vi "LabVIEW back up 05 10.vi"() -> ()   [LabVIEW 2015]
uses:
  <vilib>/DAQmx/read.llb/DAQmx Read (Analog 1D DBL NChan 1Samp).vi
  <vilib>/DAQmx/create/channels.llb/DAQmx Create Channel (AI-Voltage-Basic).vi
  <vilib>/DAQmx/miscellaneous.llb/DAQmx Fill In Error Info.vi
  Program Files/neMESYS_SDK/neMESYS LabVIEW Kit/neMESYS LabVIEW Integration Kit.lvlib
  Conor/Temp CN7500/Omega CN7500/Omega CN7500.lvlib
panel:
  in  "Empty Syringe Shut Down":bool
  out "Safety Shut Down Temp (oC)":dbl
  out "Safety Shut Down Pressure (barg)":dbl
  out "Text Read From Clipboard 5":string
  out "Read error out 5":errorcluster
  out "Write Set Point Status 2":string
  out "Error Out 5":i32
  out "Write error out 5":errorcluster
  out "Temperature":dynamicdata(graph)
  in  "Set Point (oC)":dbl
  out "Actual Temp (oC)":dbl
  out "Temp Set Point (oC)":dbl
  in  "Temperature Set Point":bool
  in  "Change New Set Points":bool
  in  "Read Set Points":bool
  in  "Test Gas Communication":bool
  out "Text Read From Clipboard":string
  out "Read error out":errorcluster
  out "Test Status":string
  out "Error Out":i32
  out "Write error out":errorcluster
  out "Text Read From Clipboard 4":string
  out "Read error out 4":errorcluster
  out "Write Set Point Status":string
  out "Error Out 4":i32
  out "Write error out 4":errorcluster
  in  "Set Point 1 (NmL/min)":dbl
  in  "Set Point 2 (NmL/min)":dbl
  in  "Set Point 3 (NmL/min)":dbl
  out "Flow Span of All Controlers (NmL/min)":dbl
  in  "Set Point 4 (NmL/min)":dbl
  out "Set Point Function":string
  out "Text Read From Clipboard 3":string
  out "Read error out 3":errorcluster
  out "Read Set Point Status":string
  out "Error Out 3":i32
  out "Write error out 3":errorcluster
  out "Text Read From Clipboard 2":string
  out "Read error out 2":errorcluster
  out "Read Flow Status":string
  out "Gas Flow 1 NmL/min":dbl
  out "Gas Flow 2 NmL/min":dbl
  out "Gas Flow 3 NmL/min":dbl
  out "Gas Flow 4 NmL/min":dbl
  out "Gas Flow rate":dynamicdata(graph)
  out "First waste string":string
  out "Rest of string 1":string
  out "First Number":string
  out "Rest of string 2":string
  out "Second Number 2":string
  out "Rest of string 3":string
  out "Third Number 3":string
  out "Rest of string 4":string
  out "Fourth Number 3":string
  out "Rest of string 5":string
  out "Error Out 2":i32
  out "Write error out 2":errorcluster
  in  "Refill 4":bool
  in  "Refill 3":bool
  in  "Refill 2":bool
  in  "Refill 1":bool
  in  "Empty 4":bool
  in  "Empty 3":bool
  in  "Empty 2":bool
  in  "Empty 1":bool
  in  "Calibrate 4":bool
  in  "Calibrate 3":bool
  in  "Calibrate 2":bool
  in  "Calibrate 1":bool
  in  "Stop Dose 4":bool
  in  "Stop Dose 3":bool
  in  "Stop Dose 2":bool
  in  "Stop Dose 1":bool
  in  "Set Level":bool
  in  "Dose Volume":bool
  in  "Generate Flow":bool
  in  "Dose Volume 4":dbl
  in  "Dose Volume 3":dbl
  in  "Dose Volume 2":dbl
  in  "Dose Volume 1":dbl
  in  "Set Level 4":dbl
  in  "Set Level 3":dbl
  in  "Set Level 2":dbl
  in  "Set Level 1":dbl
  in  "Set Flowrate 4":dbl
  in  "Set Flowrate 3":dbl
  in  "Set Flowrate 2":dbl
  in  "Set Flowrate 1":dbl
  out "Syringe Level 4":dbl
  out "Syringe Level 3":dbl
  out "Syringe Level 2":dbl
  out "Syringe Level 1":dbl
  out "Actual Flowrate 4":dbl
  out "Actual Flowrate 3":dbl
  out "Actual Flowrate 2":dbl
  out "Actual Flowrate 1":dbl
  out "Volume unit 1":string
  out "Level Max 1":dbl
  out "Flow unit 1":string
  out "Flow Max 1":dbl
  out "Number of Dosing Units":dbl
  out "Pressure 4 (barg)":dbl
  out "Pressure 3 (barg)":dbl
  out "Pressure 2 (barg)":dbl
  out "Pressure 1 (barg)":dbl
  out "Pressure 4 (PSIG)":dbl
  out "Pressure 3 (PSIG)":dbl
  out "Pressure 2 (PSIG)":dbl
  out "Pressure 1 (PSIG)":dbl
  out "Slope 4":dbl
  out "Slope 3":dbl
  out "Slope 2":dbl
  out "Intercept 4":dbl
  out "Intercept  3":dbl
  out "Intercept 2":dbl
  out "Intercept 1":dbl
  out "Slope 1":dbl
  out "Calibration File: 2":path
  in  "Clear":bool
  out "Calculated Pressure":dbl[][](graph)
  in  "stop":bool
  # "Volume and Flow units are fixed in this VI \nand we assume all syringes are identical\nBut making them a selection is easy if needed"
  # "Nemesys Pumps"
  # "Pressure Sensors"
  # "Sensor Calibration (y=psi, x=Volts) \nCalibration File is Pcal"
  # "Brooks software must be running for this to work!!!"
  # "Gas MFC"
  # "Temperature Controller"
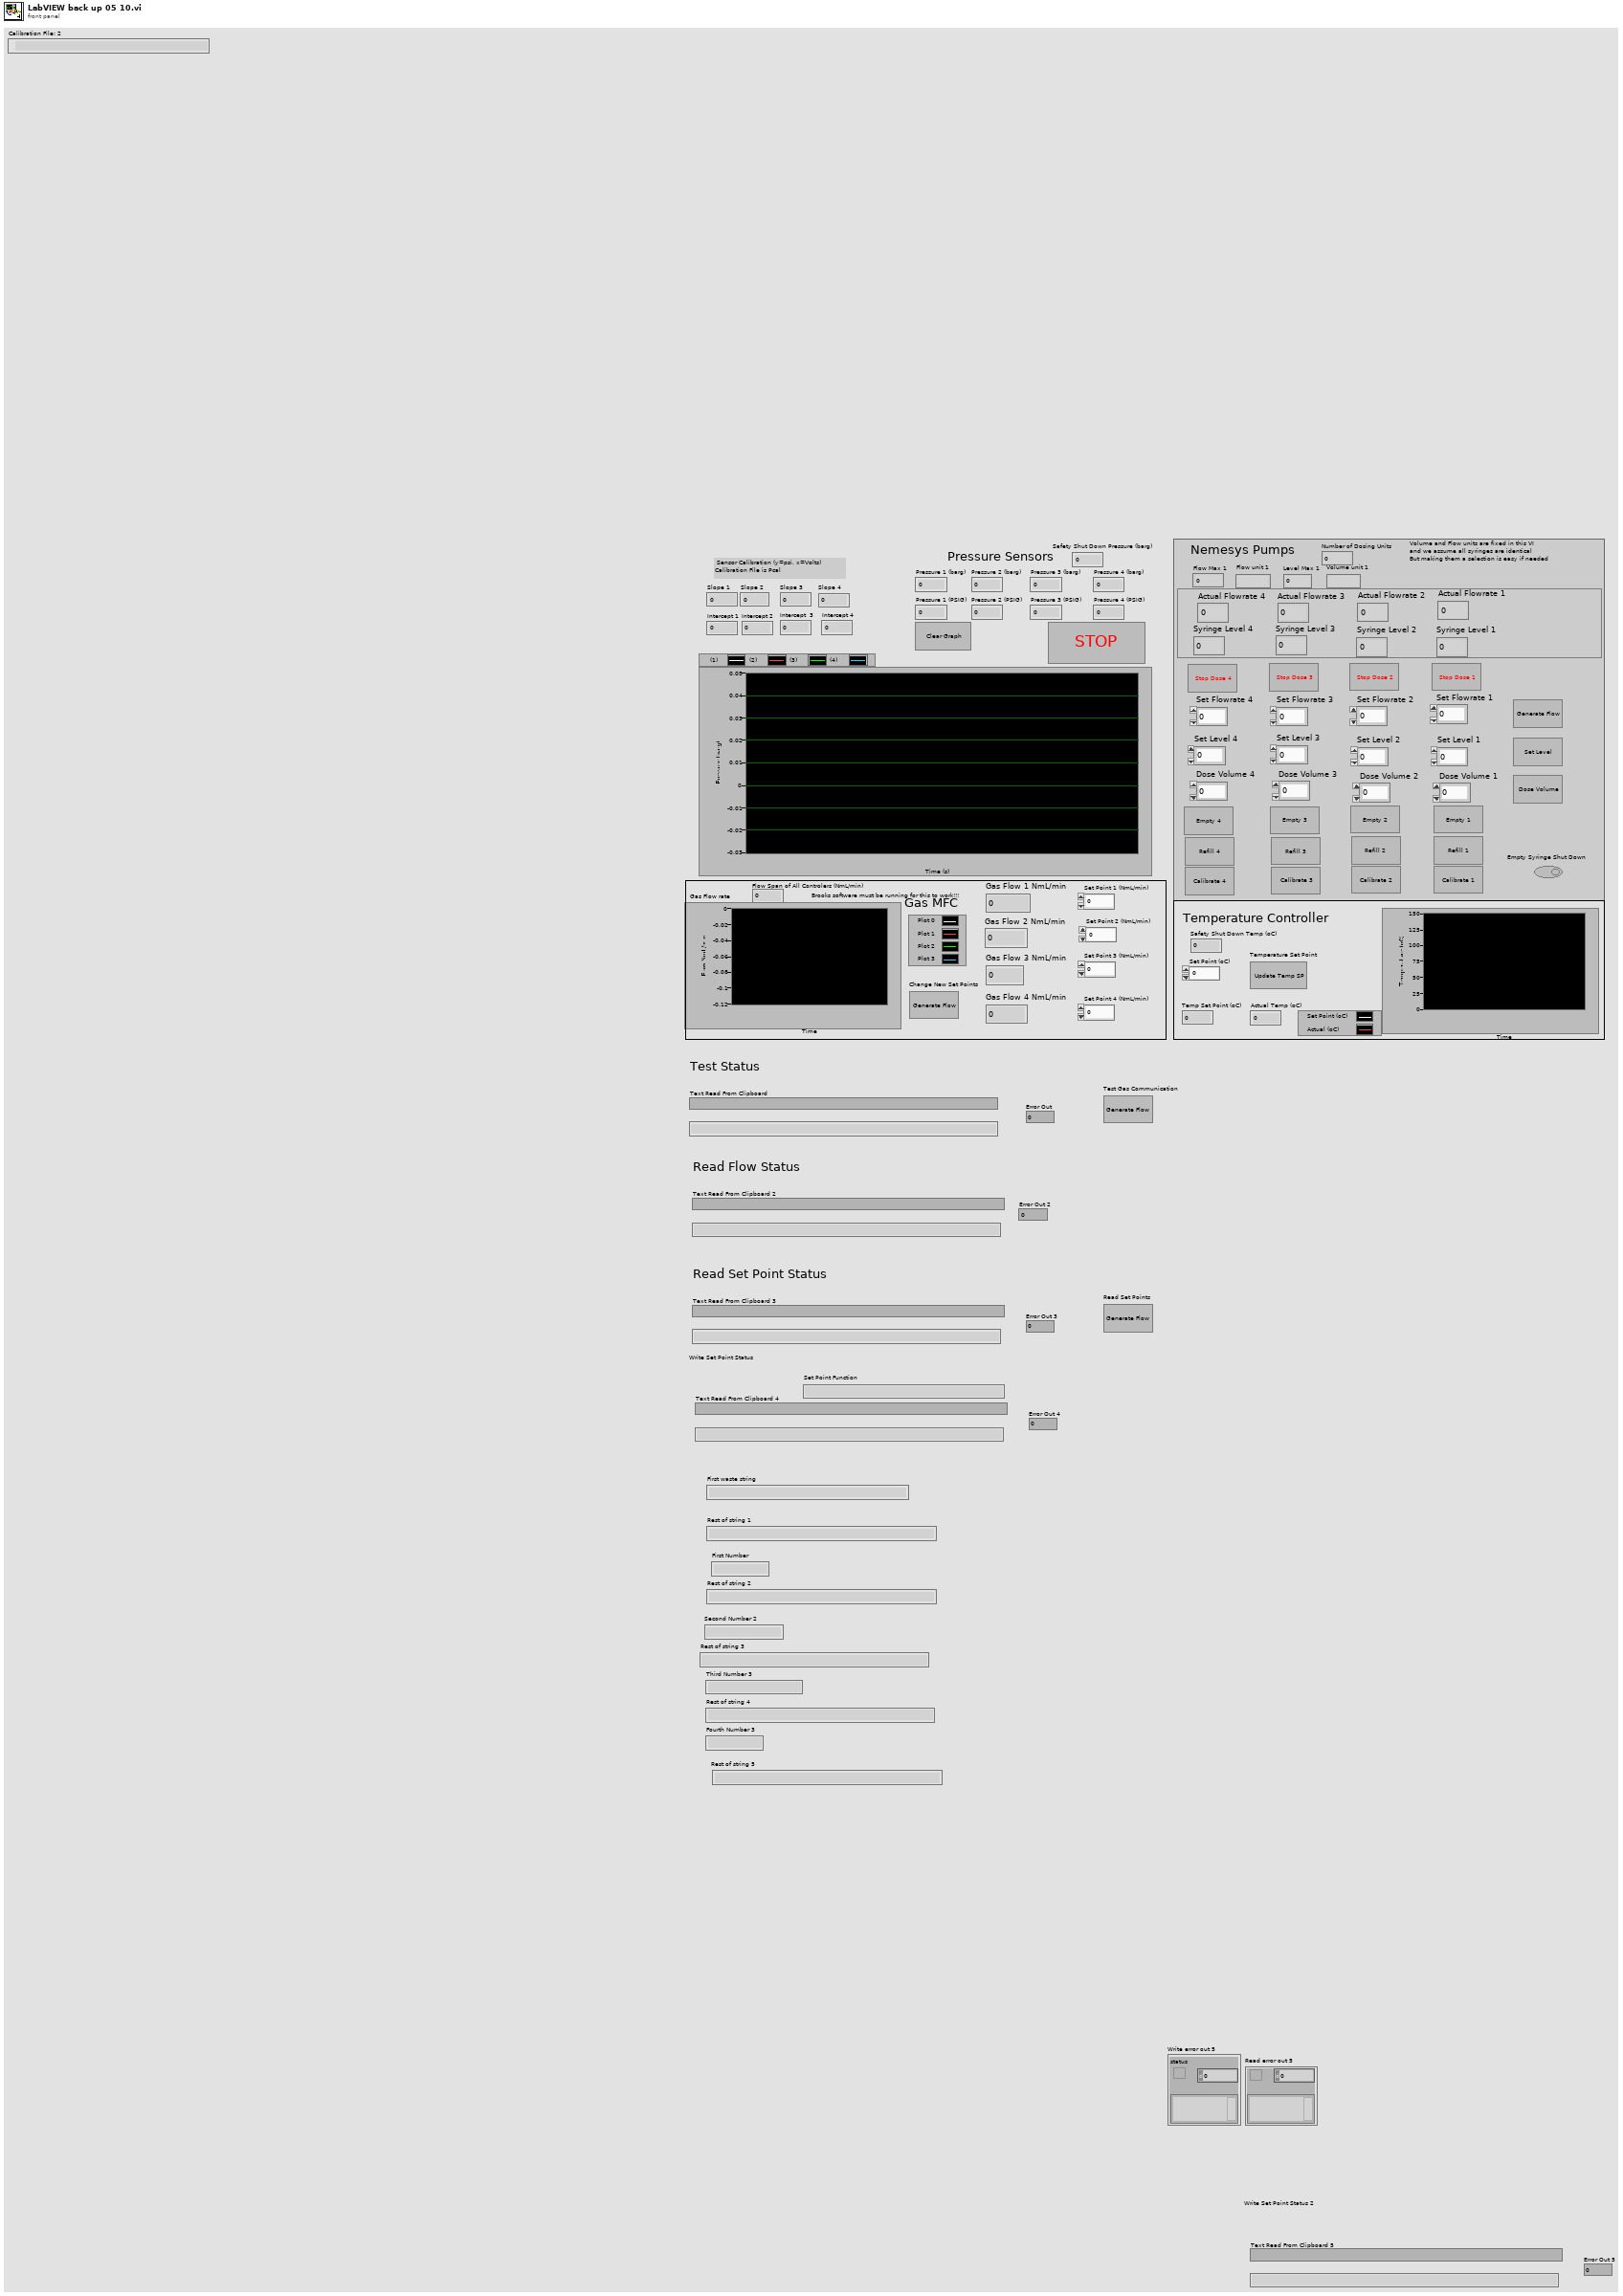
[diagram p1: front panel]
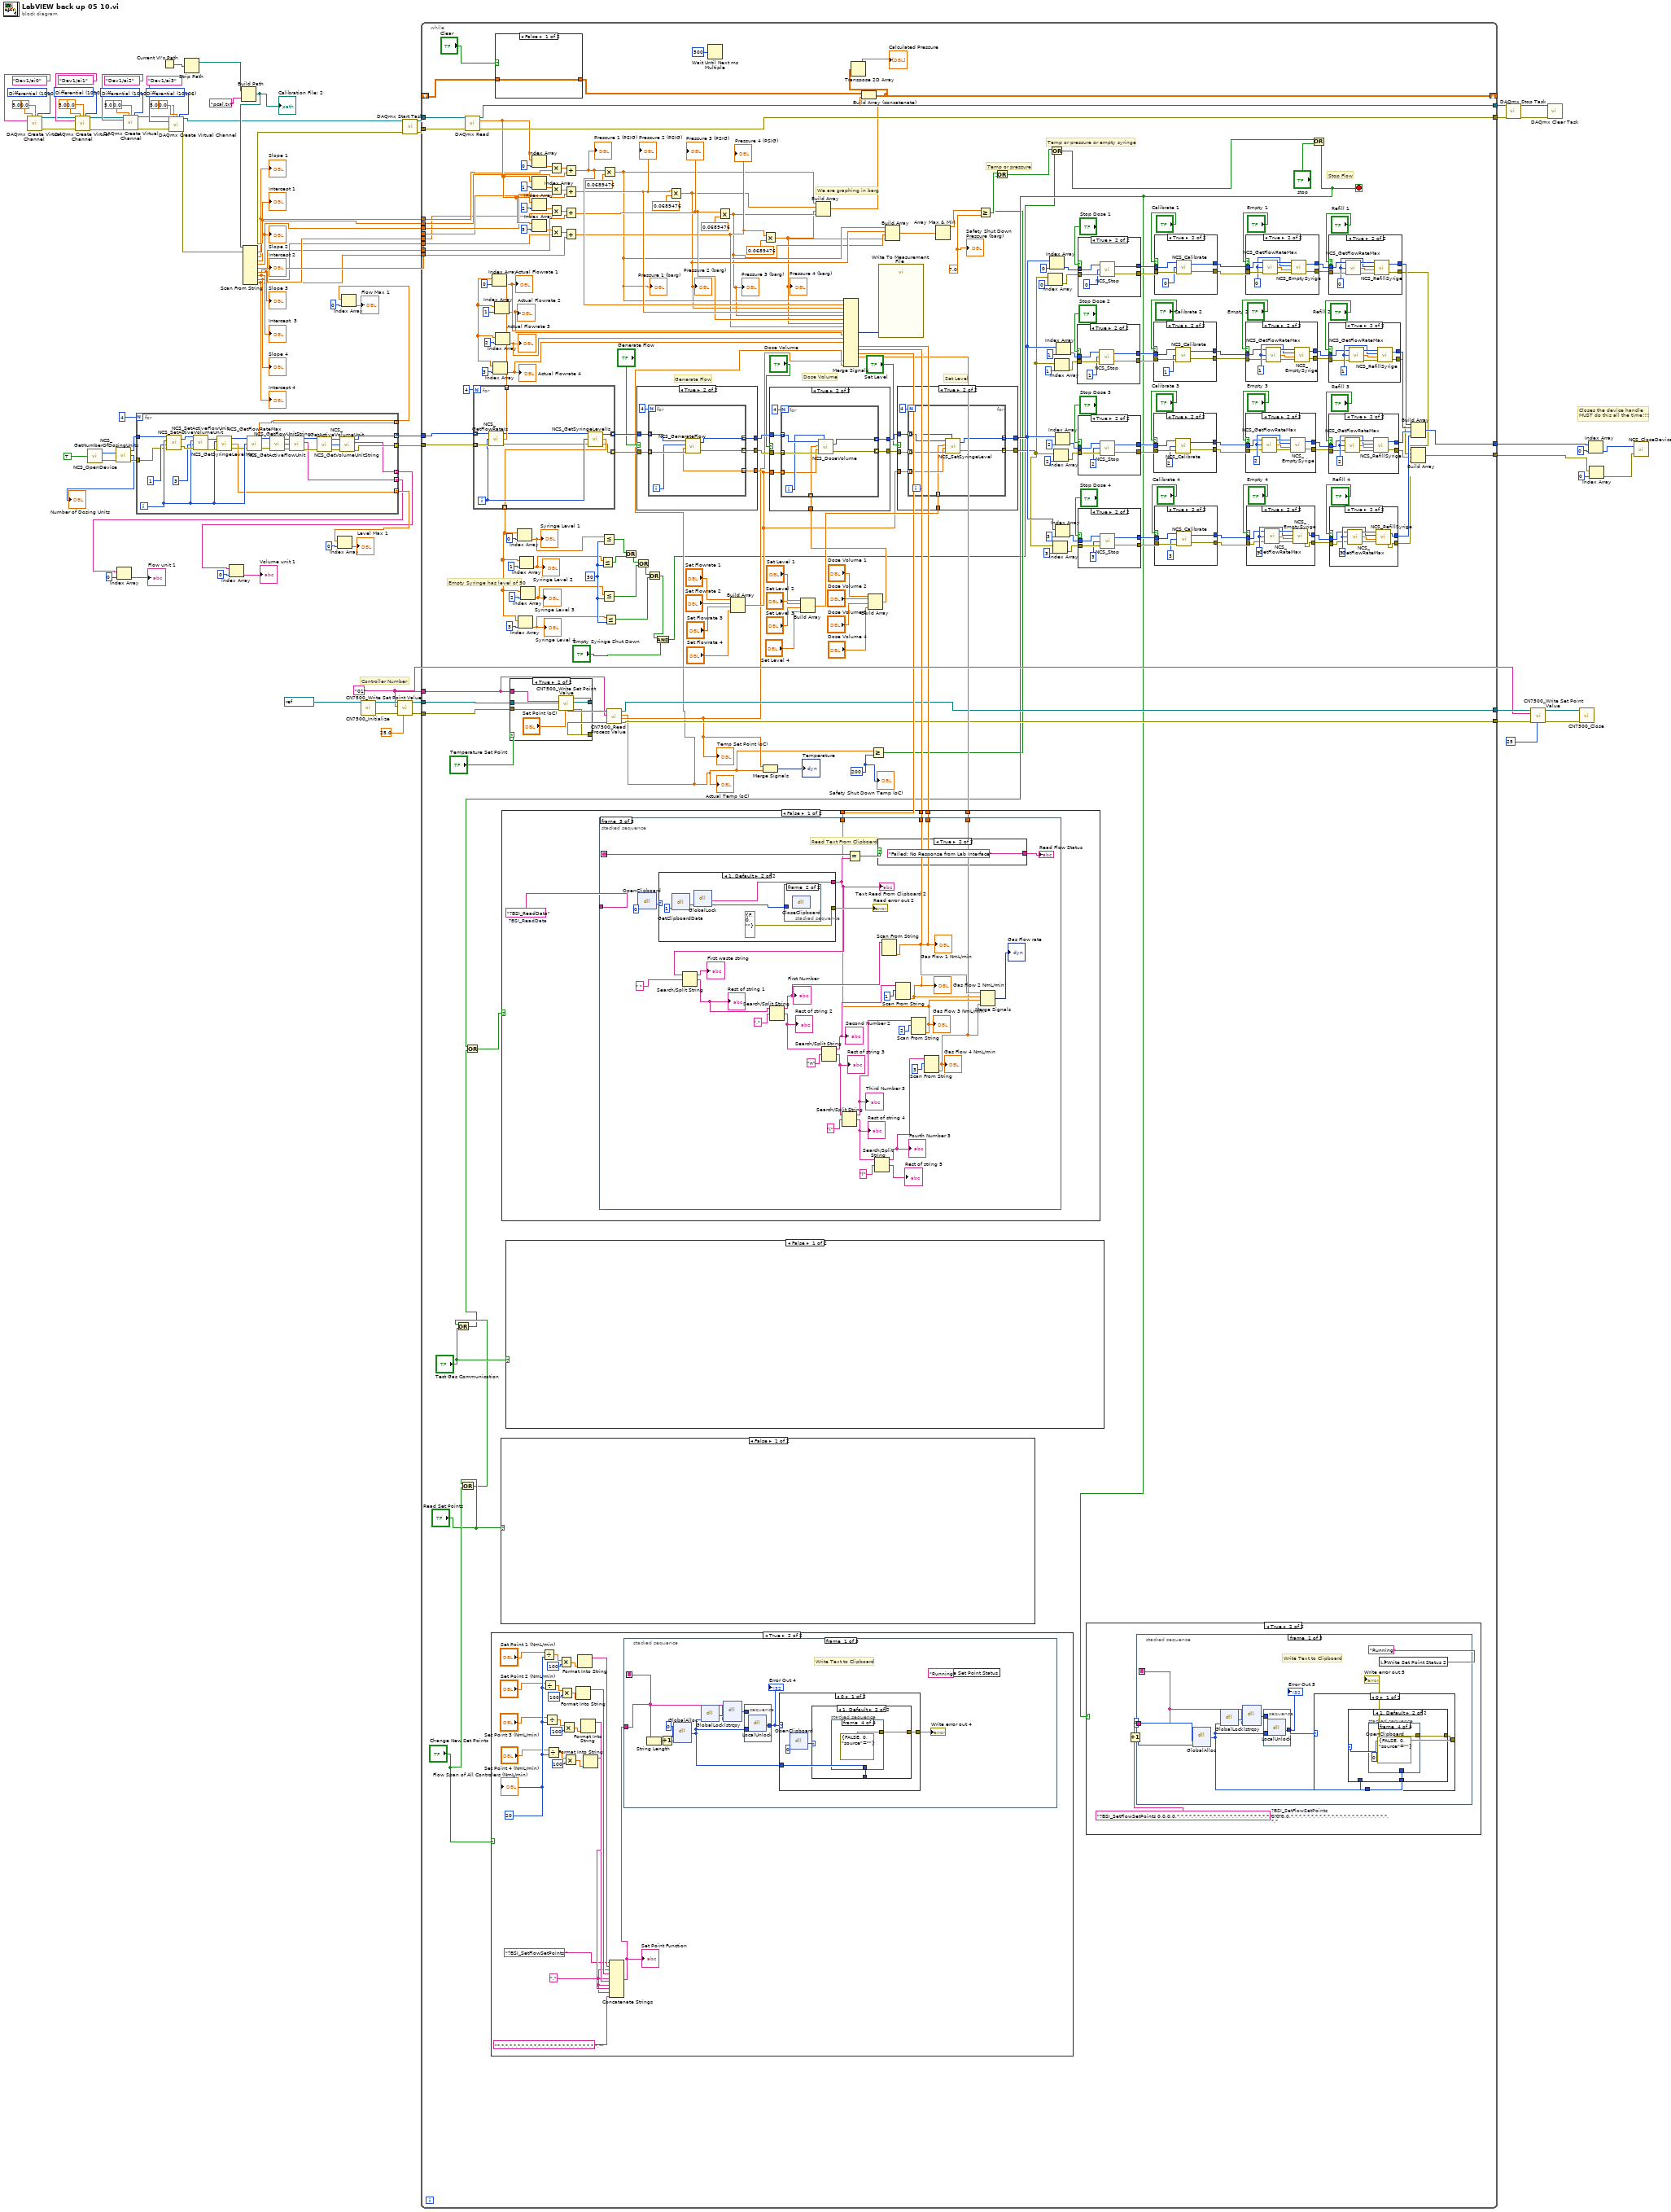
[diagram p0: block diagram]
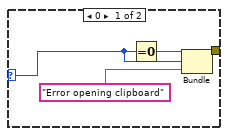
[diagram p3: hidden frame]
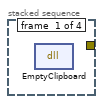
[diagram p4: hidden frame]
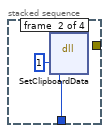
[diagram p5: hidden frame]
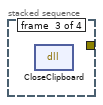
[diagram p6: hidden frame]
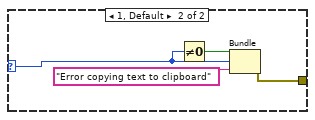
[diagram p7: hidden frame]
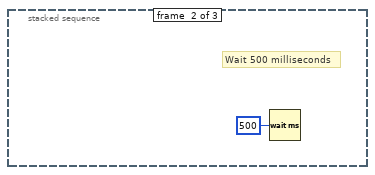
[diagram p8: hidden frame]
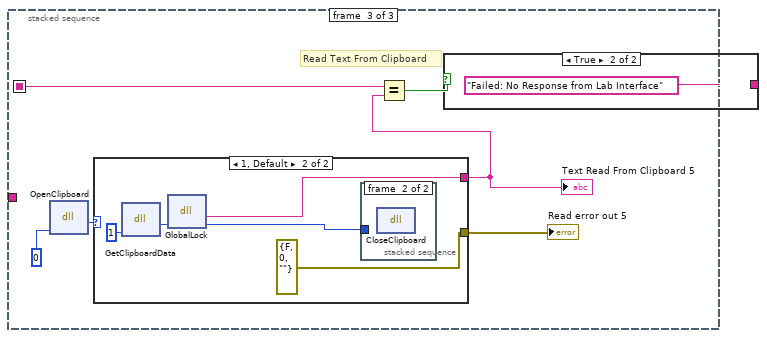
[diagram p9: hidden frame]
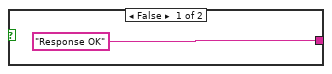
[diagram p10: hidden frame]
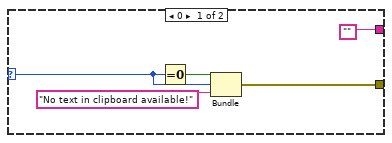
[diagram p11: hidden frame]
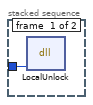
[diagram p12: hidden frame]
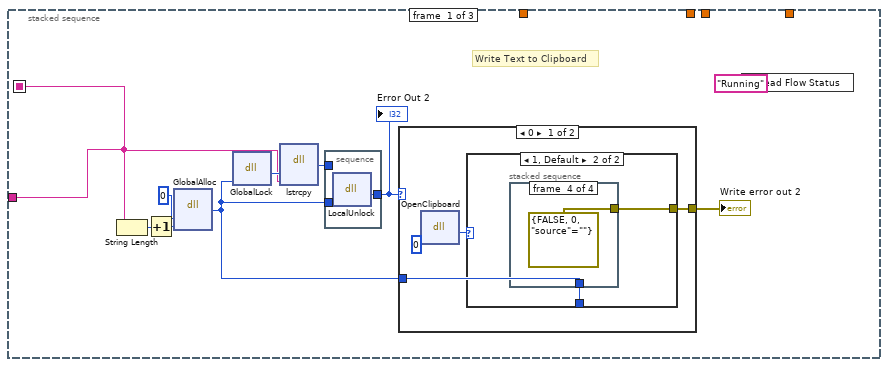
[diagram p14: hidden frame]
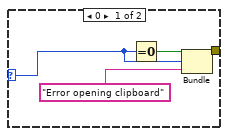
[diagram p15: hidden frame]
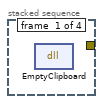
[diagram p16: hidden frame]
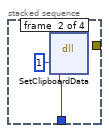
[diagram p17: hidden frame]
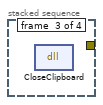
[diagram p18: hidden frame]
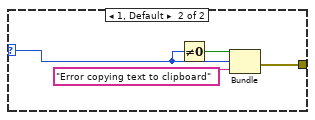
[diagram p19: hidden frame]
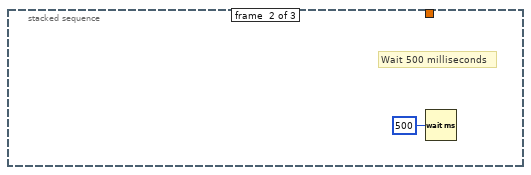
[diagram p20: hidden frame]
diagram:
  w1 = "01" ("Controller Number")
  w62 = 10106 items=["default"=-1, "RSE"=10083, "NRSE"=10078, "Differential"=10106, "Pseudodifferential"=12529] ("input terminal configuration")
  w70 = 10106 items=["default"=-1, "RSE"=10083, "NRSE"=10078, "Differential"=10106, "Pseudodifferential"=12529] ("input terminal configuration")
  w74 = 10106 items=["default"=-1, "RSE"=10083, "NRSE"=10078, "Differential"=10106, "Pseudodifferential"=12529] ("input terminal configuration")
  w82 = 10106 items=["default"=-1, "RSE"=10083, "NRSE"=10078, "Differential"=10106, "Pseudodifferential"=12529] ("input terminal configuration")
  # "Controller Number"
  # "Closes the device handle \nMUST do this all the time!!!!"
  n1 = call-poly <vilib>:"DAQmx Create Virtual Channel.vi"("maximum value"=5.0, "minimum value"=0.0, "input terminal configuration"=w62, "physical channels"=tag "Dev1/ai0") -> ("task out"=w66:refnum<k21>, "error out"=w65:errorcluster)  [unwired: 10 in]
  n2 = call-poly <vilib>:"DAQmx Create Virtual Channel.vi"("task in"=w66, "maximum value"=5.0, "minimum value"=0.0, "input terminal configuration"=w70, "physical channels"=tag "Dev1/ai1", "error in"=w65) -> ("task out"=w68:refnum<k21>, "error out"=w67:errorcluster)  [unwired: 8 in]
  n3 = call "NCS_OpenDevice.vi"("show status window"=TRUE) -> ("device handle"=w23:u32, "error out"=w22:errorcluster)
  n4 = call "NCS_GetNumberOfDosingUnits.vi"("device handle in"=w23, "error in (no error)"=w22) -> ("device handle out"=w20:u32, "number of dosing units"=→"Number of Dosing Units":u8, "error out"=w21:errorcluster)
  n5 = call-poly <vilib>:"DAQmx Create Virtual Channel.vi"("task in"=w68, "maximum value"=5.0, "minimum value"=0.0, "input terminal configuration"=w74, "physical channels"=tag "Dev1/ai2", "error in"=w67) -> ("task out"=w78:refnum<k21>, "error out"=w77:errorcluster)  [unwired: 8 in]
  n6 = for {
    N: 4 -> [_]
    tunnel: [w88] -> w37 mode=indexing
    tunnel: [w87] -> w36 mode=indexing
    tunnel: [w102] -> w33 mode=indexing
    tunnel: [w101] -> w31 mode=indexing
    tunnel: [w86] -> w28 mode=indexing
    tunnel: [w85] -> w24 mode=indexing
    tunnel: w21 -> [w84]
    tunnel: w20 -> [w83]
    i -> [w105]
    n7 = call "NCS_SetActiveVolumeUnit.vi"("error in (no error)"=w84, "active volume unit"=1, "dosingunit"=w105, "device handle in"=w83) -> ("error out"=w108:errorcluster, "device handle out"=w109:u32)
    n8 = call "NCS_SetActiveFlowUnit.vi"("error in (no error)"=w108, "active flow unit"=3, "dosingunit"=w105, "device handle in"=w109) -> ("error out"=w106:errorcluster, "device handle out"=w107:u32)
    n9 = call "NCS_GetSyringeLevelMax.vi"("error in (no error)"=w106, "dosingunit"=w105, "device handle in"=w107) -> ("error out"=w103:errorcluster, "syringe level max"=w101:dbl, "device handle out"=w104:u32)  [unwired: 1 out]
    n10 = call "NCS_GetFlowRateMax.vi"("error in (no error)"=w103, "dosingunit"=w105, "device handle in"=w104) -> ("error out"=w89:errorcluster, "flow rate max"=w102:dbl, "device handle out"=w90:u32)
    n11 = call "NCS_GetActiveFlowUnit.vi"("error in (no error)"=w89, "device handle in"=w90) -> ("error out"=w97:errorcluster, "active flow unit"=w96:u8, "device handle out"=w98:u32)  [unwired: 1 in]
    n12 = call "NCS_GetFlowUnitString.vi"("device handle in"=w98, "flow unit id"=w96, "error in (no error)"=w97) -> ("device handle out"=w93:u32, "unit string short"=w86:string, "error out"=w92:errorcluster)  [unwired: 1 out]
    n13 = call "NCS_GetActiveVolumeUnit.vi"("error in (no error)"=w92, "device handle in"=w93) -> ("error out"=w94:errorcluster, "active volume unit"=w95:u8, "device handle out"=w91:u32)  [unwired: 1 in]
    n14 = call "NCS_GetVolumeUnitString.vi"("device handle in"=w91, "volume unit id"=w95, "error in (no error)"=w94) -> ("device handle out"=w88:u32, "unit string short"=w85:string, "error out"=w87:errorcluster)  [unwired: 1 out]
  }
  n15 = Index Array(array=w28, index=0) -> (element=→"Flow unit 1":string)
  n16 = Current VI's Path() -> (path=w60:path)
  n17 = call-poly <vilib>:"DAQmx Create Virtual Channel.vi"("task in"=w78, "maximum value"=5.0, "minimum value"=0.0, "input terminal configuration"=w82, "physical channels"=tag "Dev1/ai3", "error in"=w77) -> ("task out"=w55:refnum<k21>, "error out"=w59:errorcluster)  [unwired: 8 in]
  n18 = Strip Path(path=w60) -> (stripped path=w57:path)  [unwired: 1 out]
  n19 = Index Array(array=w24, index=0) -> (element=→"Volume unit 1":string)
  n20 = Build Path(base path=w57, name or relative path="pcal.txt") -> (appended path=w58:path)
  "Calibration File: 2" <- w58
  n21 = Scan From String(w58, w59) -> (w54:errorcluster, output 1=w47:dbl, output 2=w46:dbl, output 3=w45:dbl, output 4=w44:dbl, output 5=w43:dbl, output 6=w42:dbl, output 7=w41:dbl, output 8=w40:dbl)  [unwired: 9 in, 1 out]
  "Slope 1" <- w47
  "Intercept 1" <- w46
  "Intercept 2" <- w44
  "Intercept  3" <- w42
  "Intercept 4" <- w40
  "Slope 2" <- w45
  "Slope 3" <- w43
  "Slope 4" <- w41
  n22 = Index Array(array=w31, index=0) -> (element=→"Level Max 1":dbl)
  n23 = Index Array(array=w33, index=0) -> (element=→"Flow Max 1":dbl)
  n24 = call "CN7500_Initialize.vi"("VISA resource name"=refnum<visa-resource-name> "COM7") -> ("error out"=w11:errorcluster, "VISA resource name out"=w12:refnum<visa-resource-name>)  [unwired: 9 in]
  n25 = call "CN7500_Write Set Point Value.vi"("Target Set Point Value"=25.0, "error in (no error)"=w11, "Controller Number"=w1, "VISA In"=w12) -> ("error out"=w7:errorcluster, "VISA Out"=w8:refnum<visa-resource-name>)  [unwired: 6 in]
  n26 = call <vilib>:"DAQmx Start Task.vi"("task/channels in"=w55, "error in"=w54) -> ("task out"=w53:refnum<k21>, "error out"=w52:errorcluster)  [unwired: 12 in]
  n27 = while {
    tunnel: w53 -> [w308]
    tunnel: w52 -> [w307]
    tunnel: [w306] -> w51
    tunnel: [w305] -> w50
    tunnel: w47 -> [w291]
    tunnel: w46 -> [w290]
    tunnel: w45 -> [w289]
    tunnel: w44 -> [w288]
    tunnel: w43 -> [w287]
    tunnel: w42 -> [w286]
    tunnel: w41 -> [w285]
    tunnel: w40 -> [w284]
    shift-right: [w274] -> _
    shift-left: _ -> [w278]
    tunnel: w37 -> [w266]
    tunnel: w36 -> [w265]
    tunnel: [w167] -> w17
    tunnel: [w210] -> w15
    tunnel: w8 -> [w149]
    tunnel: w7 -> [w148]
    tunnel: [w147] -> w6
    tunnel: [w146] -> w4
    tunnel: w1 -> [w143]
    stop <- w130 stop-if-true
    w125 = 50
    w128 = 200
    w133 = 7.0 ("Safety Shut Down Pressure (barg)")
    # "Temp or pressure or empty syringe"
    # "Temp or pressure"
    # "Empty Syringe has level of 50"
    # "Stop Flow"
    # "Set Level"
    # "Dose Volume"
    # "Generate Flow"
    # "We are graphing in barg"
    n28 = Or(x="Read Set Points", y="Change New Set Points") -> (x .or. y?=w155:bool)
    n29 = Or(x=w155, y="Test Gas Communication") -> (x .or. y?=w131:bool)
    n30 = call-poly <vilib>:"DAQmx Read.vi"("task/channels in"=w308, "error in"=w307) -> ("task out"=w306:refnum<k21>, "data"=w300:dbl[], "error out"=w305:errorcluster)  [unwired: 11 in]
    n31 = for {
      N: 4 -> [_]
      tunnel: w266 -> [w814] mode=indexing
      tunnel: w265 -> [w813] mode=indexing
      tunnel: [w811] -> w260 mode=indexing
      tunnel: [w808] -> w255 mode=indexing
      tunnel: [w807] -> w243 mode=indexing
      tunnel: [w806] -> w242 mode=indexing
      i -> [w812]
      n32 = call "NCS_GetFlowRateIs.vi"("error in (no error)"=w813, "dosingunit"=w812, "device handle in"=w814) -> ("error out"=w809:errorcluster, "flowrate is"=w811:dbl, "device handle out"=w810:u32)
      n33 = call "NCS_GetSyringeLevelIs.vi"("error in (no error)"=w809, "dosingunit"=w812, "device handle in"=w810) -> ("error out"=w806:errorcluster, "syringe level is"=w808:dbl, "device handle out"=w807:u32)
    }
    n34 = case shown="True" "Change New Set Points" {
      frame False {
      }
      frame True {
        w471 = 20
        w464 = ","
        n35 = Divide(x="Set Point 1 (NmL/min)", y=w471) -> (x/y=w447:dbl)
        n36 = Divide(x="Set Point 2 (NmL/min)", y=w471) -> (x/y=w449:dbl)
        n37 = Divide(x="Set Point 3 (NmL/min)", y=w471) -> (x/y=w451:dbl)
        n38 = Divide(x="Set Point 4 (NmL/min)", y=w471) -> (x/y=w453:dbl)
        n39 = Multiply(x=w447, y=100) -> (x*y=w459:dbl)
        n40 = Multiply(x=w449, y=100) -> (x*y=w460:dbl)
        n41 = Multiply(x=w451, y=100) -> (x*y=w461:dbl)
        n42 = Multiply(x=w453, y=100) -> (x*y=w462:dbl)
        n43 = Format Into String(w460) -> (resulting string=w467:string)  [unwired: 3 in, 1 out]
        n44 = Format Into String(w459) -> (resulting string=w466:string)  [unwired: 3 in, 1 out]
        n45 = Format Into String(w461) -> (resulting string=w468:string)  [unwired: 3 in, 1 out]
        n46 = Format Into String(w462) -> (resulting string=w469:string)  [unwired: 3 in, 1 out]
        n47 = Concatenate Strings("?BSI_SetFlowSetPoints ", w466, w464, w467, w464, w468, w464, w469, w464, "*,*,*,*,*,*,*,*,*,*,*,*,*,*,*,*,*,*,*,*,*,*,*,*,*,*") -> (w470:string)
        "Set Point Function" <- w470
        n48 = stacked-sequence {
          seq-local: [w472 _ _] -> [_ _ w505]
          tunnel: w470 -> [w472 _ _]
          frame #0 {
            # "Write Text to Clipboard"
            n49 = String Length(string=w472) -> (length=w481:i32)
            n50 = Increment(x=w481) -> (x+1=w477:i32)
            n51 = dll-call lib="kernel32" fn="GlobalAlloc"("Flags"=i16 0 ("Format"), "Size"=w477) -> (w476:i32)  [unwired: 5 in, 2 out]
            n52 = dll-call lib="kernel32" fn="GlobalLock"("hGlobalMemory"=w476) -> (w479:i32)  [unwired: 4 in, 2 out]
            n53 = dll-call lib="kernel32" fn="lstrcpy"("Flags"=w479, "String"=w472) -> (w478:i32)  [unwired: 5 in, 2 out]
            n54 = stacked-sequence {
              tunnel: w478 -> [_]
              tunnel: w476 -> [w500]
              tunnel: [w499] -> w475
              frame #0 {
                n55 = dll-call lib="kernel32" fn="LocalUnlock"("hGlobalMemory"=w500) -> (w499:i32)  [unwired: 4 in, 2 out]
              }
            }
            "Error Out 4" <- w475
            n56 = case shown="0" w475 {
              selector: w475 -> [_ w496]
              tunnel: w476 -> [w482 _]
              tunnel: [w483 w495] -> w474
              frame 0 {
                n57 = dll-call lib="user32" fn="OpenClipboard"("owner"=i16 0) -> (w484:i32)  [unwired: 4 in, 2 out]
                n58 = case shown="1, Default" w484 {
                  selector: w484 -> [w488 _]
                  tunnel: [w486 w491] -> w483
                  tunnel: w482 -> [_ w490]
                  frame 0 {
                    n59 = Equal To 0?(x=w488) -> (x = 0?=w489:bool)
                    n60 = Bundle(w489, w488, "source"="Error opening clipboard") -> (w486:cluster{bool, i32, "source":string})  [unwired: 1 in]
                  }
                  frame 1, Default {
                    n61 = stacked-sequence {
                      tunnel: [_ _ _ cluster{bool, i32, "source":string} {FALSE, 0, "source"=""} ("Output Element")] -> w491
                      tunnel: w490 -> [_ w492 _ _]
                      frame #0 {
                        n62 = dll-call lib="user32" fn="EmptyClipboard"() -> ()  [unwired: 4 in, 2 out]
                      }
                      frame #1 {
                        n63 = dll-call lib="user32" fn="SetClipboardData"("Format"=1, "Data"=w492) -> ()  [unwired: 6 in, 2 out]
                      }
                      frame #2 {
                        n64 = dll-call lib="user32" fn="CloseClipboard"() -> ()  [unwired: 4 in, 2 out]
                      }
                      frame #3 {
                      }
                    }
                  }
                }
              }
              frame 1, Default {
                n65 = Not Equal To 0?(x=w496) -> (x != 0?=w497:bool)
                n66 = Bundle(w497, w496, "source"="Error copying text to clipboard") -> (w495:cluster{bool, i32, "source":string})  [unwired: 1 in]
              }
            }
            "Write error out 4" <- w474
            n67 = local write "Write Set Point Status"("Running" ("Status")) -> ()
          }
          frame #1 {
            # "Wait 500 milliseconds"
            n68 = Wait (ms)(milliseconds to wait=u32 500) -> ()  [unwired: 1 out]
          }
          frame #2 {
            # "Read Text From Clipboard"
            n69 = dll-call lib="user32" fn="OpenClipboard"("owner"=i16 0) -> (w507:i32)  [unwired: 4 in, 2 out]
            n70 = case shown="1, Default" w507 {
              selector: w507 -> [w513 _]
              tunnel: ["" w518] -> w502
              tunnel: [w511 cluster{bool, i32, "source":string} {FALSE, 0, "source"=""} ("Output Element")] -> w506
              frame 0 {
                n71 = Equal To 0?(x=w513) -> (x = 0?=w514:bool)
                n72 = Bundle(w514, w513, "source"="No text in clipboard available!") -> (w511:cluster{bool, i32, "source":string})  [unwired: 1 in]
              }
              frame 1, Default {
                n73 = dll-call lib="user32" fn="GetClipboardData"("uFormat"=1 ("hGlobalMemory")) -> (w519:i32)  [unwired: 4 in, 2 out]
                n74 = dll-call lib="kernel32" fn="GlobalLock"("hGlobalMemory"=w519) -> (w518:string, "hGlobalMemory"=w516:i32)  [unwired: 3 in, 2 out]
                n75 = stacked-sequence {
                  tunnel: w516 -> [w521 _]
                  frame #0 {
                    n76 = dll-call lib="kernel32" fn="LocalUnlock"("hGlobalMemory"=w521) -> ()  [unwired: 5 in, 2 out]
                  }
                  frame #1 {
                    n77 = dll-call lib="user32" fn="CloseClipboard"() -> ()  [unwired: 4 in, 2 out]
                  }
                }
              }
            }
            "Text Read From Clipboard 4" <- w502
            "Read error out 4" <- w506
            n78 = Equal?(x=w505, y=w502) -> (x = y?=w504:bool)
            n79 = case shown="True" w504 {
              tunnel: ["Response OK" "Failed: No Response from Lab Interface"] -> w503
              frame False {
              }
              frame True {
              }
            }
            "Write Set Point Status" <- w503
          }
        }
        "Flow Span of All Controlers (NmL/min)" <- w471
      }
    }
    n80 = Index Array(array=w260, index=0) -> (element=w162:dbl)
    "Actual Flowrate 1" <- w162
    n81 = Index Array(array=w260, index=3) -> (element=w159:dbl)
    "Actual Flowrate 4" <- w159
    n82 = Index Array(array=w260, index=1) -> (element=w161:dbl)
    "Actual Flowrate 2" <- w161
    n83 = case shown="False" "Clear" {
      tunnel: w278 -> [w815 _]
      tunnel: [w815 w816] -> w276
      frame False {
      }
      frame True {
        n84 = Initialize Array(0.0 ("element"), 1 ("dimension size"), 4 ("dimension size")) -> (w816:dbl[][])
      }
    }
    n85 = Index Array(array=w260, index=2) -> (element=w160:dbl)
    "Actual Flowrate 3" <- w160
    n86 = case shown="False" "Read Set Points" {
      frame False {
      }
      frame True {
        w522 = "?BSI_ReadFlowSetPoints"  # ?BSI_ReadFlowSetPoints
        n87 = stacked-sequence {
          seq-local: [w523 _ _] -> [_ _ w556]
          tunnel: w522 -> [w523 _ _]
          frame #0 {
            # "Write Text to Clipboard"
            n88 = String Length(string=w523) -> (length=w532:i32)
            n89 = Increment(x=w532) -> (x+1=w528:i32)
            n90 = dll-call lib="kernel32" fn="GlobalAlloc"("Flags"=i16 0 ("Format"), "Size"=w528) -> (w527:i32)  [unwired: 5 in, 2 out]
            n91 = dll-call lib="kernel32" fn="GlobalLock"("hGlobalMemory"=w527) -> (w530:i32)  [unwired: 4 in, 2 out]
            n92 = dll-call lib="kernel32" fn="lstrcpy"("Flags"=w530, "String"=w523) -> (w529:i32)  [unwired: 5 in, 2 out]
            n93 = stacked-sequence {
              tunnel: w529 -> [_]
              tunnel: w527 -> [w551]
              tunnel: [w550] -> w526
              frame #0 {
                n94 = dll-call lib="kernel32" fn="LocalUnlock"("hGlobalMemory"=w551) -> (w550:i32)  [unwired: 4 in, 2 out]
              }
            }
            "Error Out 3" <- w526
            n95 = case shown="0" w526 {
              selector: w526 -> [_ w547]
              tunnel: w527 -> [w533 _]
              tunnel: [w534 w546] -> w525
              frame 0 {
                n96 = dll-call lib="user32" fn="OpenClipboard"("owner"=i16 0) -> (w535:i32)  [unwired: 4 in, 2 out]
                n97 = case shown="1, Default" w535 {
                  selector: w535 -> [w539 _]
                  tunnel: [w537 w542] -> w534
                  tunnel: w533 -> [_ w541]
                  frame 0 {
                    n98 = Equal To 0?(x=w539) -> (x = 0?=w540:bool)
                    n99 = Bundle(w540, w539, "source"="Error opening clipboard") -> (w537:cluster{bool, i32, "source":string})  [unwired: 1 in]
                  }
                  frame 1, Default {
                    n100 = stacked-sequence {
                      tunnel: [_ _ _ cluster{bool, i32, "source":string} {FALSE, 0, "source"=""} ("Output Element")] -> w542
                      tunnel: w541 -> [_ w543 _ _]
                      frame #0 {
                        n101 = dll-call lib="user32" fn="EmptyClipboard"() -> ()  [unwired: 4 in, 2 out]
                      }
                      frame #1 {
                        n102 = dll-call lib="user32" fn="SetClipboardData"("Format"=1, "Data"=w543) -> ()  [unwired: 6 in, 2 out]
                      }
                      frame #2 {
                        n103 = dll-call lib="user32" fn="CloseClipboard"() -> ()  [unwired: 4 in, 2 out]
                      }
                      frame #3 {
                      }
                    }
                  }
                }
              }
              frame 1, Default {
                n104 = Not Equal To 0?(x=w547) -> (x != 0?=w548:bool)
                n105 = Bundle(w548, w547, "source"="Error copying text to clipboard") -> (w546:cluster{bool, i32, "source":string})  [unwired: 1 in]
              }
            }
            "Write error out 3" <- w525
            n106 = local write "Read Set Point Status"("Running" ("Status")) -> ()
          }
          frame #1 {
            # "Wait 500 milliseconds"
            n107 = Wait (ms)(milliseconds to wait=u32 500) -> ()  [unwired: 1 out]
          }
          frame #2 {
            # "Read Text From Clipboard"
            n108 = dll-call lib="user32" fn="OpenClipboard"("owner"=i16 0) -> (w558:i32)  [unwired: 4 in, 2 out]
            n109 = case shown="1, Default" w558 {
              selector: w558 -> [w564 _]
              tunnel: ["" w569] -> w553
              tunnel: [w562 cluster{bool, i32, "source":string} {FALSE, 0, "source"=""} ("Output Element")] -> w557
              frame 0 {
                n110 = Equal To 0?(x=w564) -> (x = 0?=w565:bool)
                n111 = Bundle(w565, w564, "source"="No text in clipboard available!") -> (w562:cluster{bool, i32, "source":string})  [unwired: 1 in]
              }
              frame 1, Default {
                n112 = dll-call lib="user32" fn="GetClipboardData"("uFormat"=1 ("hGlobalMemory")) -> (w570:i32)  [unwired: 4 in, 2 out]
                n113 = dll-call lib="kernel32" fn="GlobalLock"("hGlobalMemory"=w570) -> (w569:string, "hGlobalMemory"=w567:i32)  [unwired: 3 in, 2 out]
                n114 = stacked-sequence {
                  tunnel: w567 -> [w572 _]
                  frame #0 {
                    n115 = dll-call lib="kernel32" fn="LocalUnlock"("hGlobalMemory"=w572) -> ()  [unwired: 5 in, 2 out]
                  }
                  frame #1 {
                    n116 = dll-call lib="user32" fn="CloseClipboard"() -> ()  [unwired: 4 in, 2 out]
                  }
                }
              }
            }
            "Text Read From Clipboard 3" <- w553
            "Read error out 3" <- w557
            n117 = Equal?(x=w556, y=w553) -> (x = y?=w555:bool)
            n118 = case shown="True" w555 {
              tunnel: ["Response OK" "Failed: No Response from Lab Interface"] -> w554
              frame False {
              }
              frame True {
              }
            }
            "Read Set Point Status" <- w554
          }
        }
      }
    }
    n119 = case shown="False" "Test Gas Communication" {
      frame False {
      }
      frame True {
        w573 = "?BSI_Test"  # ?BSI_Test
        n120 = stacked-sequence {
          seq-local: [w574 _ _] -> [_ _ w607]
          tunnel: w573 -> [w574 _ _]
          frame #0 {
            # "Write Text to Clipboard"
            n121 = String Length(string=w574) -> (length=w583:i32)
            n122 = Increment(x=w583) -> (x+1=w579:i32)
            n123 = dll-call lib="kernel32" fn="GlobalAlloc"("Flags"=i16 0 ("Format"), "Size"=w579) -> (w578:i32)  [unwired: 5 in, 2 out]
            n124 = dll-call lib="kernel32" fn="GlobalLock"("hGlobalMemory"=w578) -> (w581:i32)  [unwired: 4 in, 2 out]
            n125 = dll-call lib="kernel32" fn="lstrcpy"("Flags"=w581, "String"=w574) -> (w580:i32)  [unwired: 5 in, 2 out]
            n126 = stacked-sequence {
              tunnel: w580 -> [_]
              tunnel: w578 -> [w602]
              tunnel: [w601] -> w577
              frame #0 {
                n127 = dll-call lib="kernel32" fn="LocalUnlock"("hGlobalMemory"=w602) -> (w601:i32)  [unwired: 4 in, 2 out]
              }
            }
            "Error Out" <- w577
            n128 = case shown="1, Default" w577 {
              selector: w577 -> [_ w598]
              tunnel: w578 -> [w584 _]
              tunnel: [w585 w597] -> w576
              frame 0 {
                n129 = dll-call lib="user32" fn="OpenClipboard"("owner"=i16 0) -> (w586:i32)  [unwired: 4 in, 2 out]
                n130 = case shown="0" w586 {
                  selector: w586 -> [w590 _]
                  tunnel: [w588 w593] -> w585
                  tunnel: w584 -> [_ w592]
                  frame 0 {
                    n131 = Equal To 0?(x=w590) -> (x = 0?=w591:bool)
                    n132 = Bundle(w591, w590, "source"="Error opening clipboard") -> (w588:cluster{bool, i32, "source":string})  [unwired: 1 in]
                  }
                  frame 1, Default {
                    n133 = stacked-sequence {
                      tunnel: [_ _ _ cluster{bool, i32, "source":string} {FALSE, 0, "source"=""} ("Output Element")] -> w593
                      tunnel: w592 -> [_ w594 _ _]
                      frame #0 {
                        n134 = dll-call lib="user32" fn="EmptyClipboard"() -> ()  [unwired: 4 in, 2 out]
                      }
                      frame #1 {
                        n135 = dll-call lib="user32" fn="SetClipboardData"("Format"=1, "Data"=w594) -> ()  [unwired: 6 in, 2 out]
                      }
                      frame #2 {
                        n136 = dll-call lib="user32" fn="CloseClipboard"() -> ()  [unwired: 4 in, 2 out]
                      }
                      frame #3 {
                      }
                    }
                  }
                }
              }
              frame 1, Default {
                n137 = Not Equal To 0?(x=w598) -> (x != 0?=w599:bool)
                n138 = Bundle(w599, w598, "source"="Error copying text to clipboard") -> (w597:cluster{bool, i32, "source":string})  [unwired: 1 in]
              }
            }
            "Write error out" <- w576
            n139 = local write "Test Status"("Running" ("Status")) -> ()
          }
          frame #1 {
            # "Wait 500 milliseconds"
            n140 = Wait (ms)(milliseconds to wait=u32 500) -> ()  [unwired: 1 out]
          }
          frame #2 {
            # "Read Text From Clipboard"
            n141 = dll-call lib="user32" fn="OpenClipboard"("owner"=i16 0) -> (w609:i32)  [unwired: 4 in, 2 out]
            n142 = case shown="1, Default" w609 {
              selector: w609 -> [w615 _]
              tunnel: ["" w620] -> w604
              tunnel: [w613 cluster{bool, i32, "source":string} {FALSE, 0, "source"=""} ("Output Element")] -> w608
              frame 0 {
                n143 = Equal To 0?(x=w615) -> (x = 0?=w616:bool)
                n144 = Bundle(w616, w615, "source"="No text in clipboard available!") -> (w613:cluster{bool, i32, "source":string})  [unwired: 1 in]
              }
              frame 1, Default {
                n145 = dll-call lib="user32" fn="GetClipboardData"("uFormat"=1 ("hGlobalMemory")) -> (w621:i32)  [unwired: 4 in, 2 out]
                n146 = dll-call lib="kernel32" fn="GlobalLock"("hGlobalMemory"=w621) -> (w620:string, "hGlobalMemory"=w618:i32)  [unwired: 3 in, 2 out]
                n147 = stacked-sequence {
                  tunnel: w618 -> [w623 _]
                  frame #0 {
                    n148 = dll-call lib="kernel32" fn="LocalUnlock"("hGlobalMemory"=w623) -> ()  [unwired: 5 in, 2 out]
                  }
                  frame #1 {
                    n149 = dll-call lib="user32" fn="CloseClipboard"() -> ()  [unwired: 4 in, 2 out]
                  }
                }
              }
            }
            "Text Read From Clipboard" <- w604
            "Read error out" <- w608
            n150 = Equal?(x=w607, y=w604) -> (x = y?=w606:bool)
            n151 = case shown="True" w606 {
              tunnel: ["Response OK" "Failed: No Response from Lab Interface"] -> w605
              frame False {
              }
              frame True {
              }
            }
            "Test Status" <- w605
          }
        }
      }
    }
    n152 = case shown="True" "Temperature Set Point" {
      tunnel: w149 -> [w361 w367]
      tunnel: w148 -> [w360 w366]
      tunnel: [w361 w365] -> w144
      tunnel: [w360 w364] -> w145
      tunnel: w143 -> [_ w363]
      frame False {
      }
      frame True {
        n153 = call "CN7500_Write Set Point Value.vi"("Target Set Point Value"="Set Point (oC)", "error in (no error)"=w366, "Controller Number"=w363, "VISA In"=w367) -> ("error out"=w364:errorcluster, "VISA Out"=w365:refnum<visa-resource-name>)  [unwired: 6 in]
      }
    }
    n154 = Index Array(array=w255, index=0) -> (element=w124:dbl)
    "Syringe Level 1" <- w124
    n155 = Index Array(array=w255, index=3) -> (element=w121:dbl)
    "Syringe Level 4" <- w121
    n156 = Index Array(array=w255, index=1) -> (element=w123:dbl)
    "Syringe Level 2" <- w123
    n157 = Index Array(array=w255, index=2) -> (element=w122:dbl)
    "Syringe Level 3" <- w122
    n158 = Index Array(array=w300, index=0) -> (element=w295:dbl)
    n159 = Index Array(array=w300, index=1) -> (element=w294:dbl)
    n160 = Index Array(array=w300, index=2) -> (element=w293:dbl)
    n161 = Index Array(array=w300, index=3) -> (element=w292:dbl)
    n162 = Multiply(x=w295, y=w291) -> (x*y=w299:dbl)
    n163 = Multiply(x=w294, y=w289) -> (x*y=w298:dbl)
    n164 = Multiply(x=w293, y=w287) -> (x*y=w297:dbl)
    n165 = Multiply(x=w292, y=w285) -> (x*y=w296:dbl)
    n166 = Add(x=w299, y=w290) -> (x+y=w271:dbl)
    "Pressure 1 (PSIG)" <- w271
    n167 = Add(x=w298, y=w288) -> (x+y=w270:dbl)
    "Pressure 2 (PSIG)" <- w270
    n168 = Add(x=w297, y=w286) -> (x+y=w269:dbl)
    "Pressure 3 (PSIG)" <- w269
    n169 = Add(x=w296, y=w284) -> (x+y=w268:dbl)
    "Pressure 4 (PSIG)" <- w268
    n170 = Less Or Equal?(x=w123, y=w125) -> (x <= y?=w120:bool)
    n171 = Less Or Equal?(x=w124, y=w125) -> (x <= y?=w119:bool)
    n172 = Less Or Equal?(x=w122, y=w125) -> (x <= y?=w117:bool)
    n173 = Multiply(x=w271, y=0.0689476) -> (x*y=w140:dbl)
    "Pressure 1 (barg)" <- w140
    n174 = Less Or Equal?(x=w121, y=w125) -> (x <= y?=w115:bool)
    n175 = call "CN7500_Read Process Value.vi"("error in (no error)"=w145, "Controller Number"=w143, "VISA In"=w144) -> ("error out"=w146:errorcluster, "Set Point Value"=w141:dbl, "Process Value"=w129:dbl, "VISA Out"=w147:refnum<visa-resource-name>)  [unwired: 5 in]
    "Temp Set Point (oC)" <- w141
    "Actual Temp (oC)" <- w129
    n176 = Or(x=w119, y=w120) -> (x .or. y?=w118:bool)
    n177 = Or(x=w118, y=w117) -> (x .or. y?=w116:bool)
    n178 = Or(x=w116, y=w115) -> (x .or. y?=w111:bool)
    n179 = And(x=w111, y="Empty Syringe Shut Down") -> (x .and. y?=w112:bool)
    n180 = Multiply(x=w270, y=0.0689476) -> (x*y=w139:dbl)
    "Pressure 2 (barg)" <- w139
    n181 = Wait Until Next ms Multiple(millisecond multiple=u32 500) -> ()  [unwired: 1 out]
    n182 = Multiply(x=w269, y=0.0689476) -> (x*y=w138:dbl)
    "Pressure 3 (barg)" <- w138
    n183 = Build Array("Set Flowrate 1", "Set Flowrate 2", "Set Flowrate 3", "Set Flowrate 4") -> (w233:dbl[])
    n184 = case shown="True" "Generate Flow" {
      tunnel: w243 -> [w793 w798]
      tunnel: w242 -> [w792 w797]
      tunnel: [w792 w796] -> w238
      tunnel: [w793 w795] -> w239
      tunnel: w233 -> [_ w794]
      frame False {
      }
      frame True {
        n185 = for {
          N: 4 -> [_]
          tunnel: w798 -> [w805] mode=indexing
          tunnel: w797 -> [w804] mode=indexing
          tunnel: [w803] -> w796 mode=indexing
          tunnel: [w802] -> w795 mode=indexing
          tunnel: w794 -> [w800] mode=indexing
          i -> [w801]
          n186 = call "NCS_GenerateFlow.vi"("error in (no error)"=w804, "flowrate"=w800, "dosingunit"=w801, "device handle in"=w805) -> ("error out"=w803:errorcluster, "device handle out"=w802:u32)
        }
      }
    }
    n187 = Multiply(x=w268, y=0.0689476) -> (x*y=w137:dbl)
    "Pressure 4 (barg)" <- w137
    n188 = Merge Signals(w141, w129) -> (→"Temperature":dynamicdata)
    n189 = Build Array("Set Level 1", "Set Level 2", "Set Level 3", "Set Level 4") -> (w234:dbl[])
    n190 = Build Array(w140, w139, w138, w137) -> (w277:dbl[])
    n191 = Build Array (concatenate)(w276, w277) -> (w274:dbl[][])
    n192 = Transpose 2D Array(2D array=w274) -> (transposed array=→"Calculated Pressure":dbl[][])
    n193 = Build Array("Dose Volume 1", "Dose Volume 2", "Dose Volume 3", "Dose Volume 4") -> (w237:dbl[])
    n194 = case shown="True" "Dose Volume" {
      tunnel: w239 -> [w777 w783]
      tunnel: w238 -> [w776 w782]
      tunnel: [w776 w781] -> w235
      tunnel: [w777 w780] -> w236
      tunnel: w233 -> [_ w779]
      tunnel: w237 -> [_ w778]
      frame False {
      }
      frame True {
        n195 = for {
          N: 4 -> [_]
          tunnel: w783 -> [w788] mode=indexing
          tunnel: w782 -> [w791] mode=indexing
          tunnel: [w790] -> w781 mode=indexing
          tunnel: [w789] -> w780 mode=indexing
          tunnel: w779 -> [w786] mode=indexing
          tunnel: w778 -> [w785] mode=indexing
          i -> [w787]
          n196 = call "NCS_DoseVolume.vi"("device handle in"=w788, "volume"=w785, "flowrate"=w786, "error in (no error)"=w791, "dosingunit"=w787) -> ("device handle out"=w789:u32, "error out"=w790:errorcluster)
        }
      }
    }
    n197 = Greater Or Equal?(x=w129, y=w128) -> (x >= y?=w126:bool)
    n198 = Build Array(w140, w139, w138, w137) -> (w136:dbl[])
    n199 = case shown="True" "Set Level" {
      tunnel: w236 -> [w761 w767]
      tunnel: w235 -> [w760 w766]
      tunnel: [w760 w765] -> w208
      tunnel: [w761 w764] -> w209
      tunnel: w233 -> [_ w763]
      tunnel: w234 -> [_ w762]
      frame False {
      }
      frame True {
        n200 = for {
          N: 4 -> [_]
          tunnel: w767 -> [w772] mode=indexing
          tunnel: w766 -> [w775] mode=indexing
          tunnel: [w774] -> w765 mode=indexing
          tunnel: [w773] -> w764 mode=indexing
          tunnel: w763 -> [w770] mode=indexing
          tunnel: w762 -> [w769] mode=indexing
          i -> [w771]
          n201 = call "NCS_SetSyringeLevel.vi"("device handle in"=w772, "volume"=w769, "flowrate"=w770, "error in (no error)"=w775, "dosingunit"=w771) -> ("device handle out"=w773:u32, "error out"=w774:errorcluster)
        }
      }
    }
    n202 = Array Max & Min(array=w136) -> (max value=w135:dbl)  [unwired: 3 out]
    n203 = Greater Or Equal?(x=w135, y=w133) -> (x >= y?=w127:bool)
    n204 = Or(x=w127, y=w126) -> (x .or. y?=w113:bool)
    n205 = Index Array(array=w208, index=0) -> (element=w221:errorcluster)
    n206 = Or(x=w113, y=w112) -> (x .or. y?=w114:bool)
    n207 = Index Array(array=w209, index=0) -> (element=w222:u32)
    n208 = Index Array(array=w208, index=3) -> (element=w211:errorcluster)
    n209 = Index Array(array=w208, index=2) -> (element=w213:errorcluster)
    n210 = Index Array(array=w208, index=1) -> (element=w215:errorcluster)
    n211 = Index Array(array=w209, index=3) -> (element=w212:u32)
    n212 = Index Array(array=w209, index=2) -> (element=w214:u32)
    n213 = Index Array(array=w209, index=1) -> (element=w216:u32)
    n214 = case shown="True" "Stop Dose 2" {
      tunnel: w216 -> [w747 w752]
      tunnel: w215 -> [w746 w751]
      tunnel: [w747 w750] -> w201
      tunnel: [w746 w749] -> w200
      frame False {
      }
      frame True {
        n215 = call "NCS_Stop.vi"("error in (no error)"=w751, "dosingunit"=1, "device handle in"=w752) -> ("error out"=w749:errorcluster, "device handle out"=w750:u32)
      }
    }
    n216 = case shown="True" "Stop Dose 1" {
      tunnel: w222 -> [w754 w759]
      tunnel: w221 -> [w753 w758]
      tunnel: [w754 w757] -> w203
      tunnel: [w753 w756] -> w202
      frame False {
      }
      frame True {
        n217 = call "NCS_Stop.vi"("error in (no error)"=w758, "dosingunit"=0, "device handle in"=w759) -> ("error out"=w756:errorcluster, "device handle out"=w757:u32)
      }
    }
    n218 = case shown="True" "Stop Dose 3" {
      tunnel: w214 -> [w740 w745]
      tunnel: w213 -> [w739 w744]
      tunnel: [w740 w743] -> w199
      tunnel: [w739 w742] -> w198
      frame False {
      }
      frame True {
        n219 = call "NCS_Stop.vi"("error in (no error)"=w744, "dosingunit"=2, "device handle in"=w745) -> ("error out"=w742:errorcluster, "device handle out"=w743:u32)
      }
    }
    n220 = case shown="True" "Stop Dose 4" {
      tunnel: w212 -> [w733 w738]
      tunnel: w211 -> [w732 w737]
      tunnel: [w733 w736] -> w197
      tunnel: [w732 w735] -> w196
      frame False {
      }
      frame True {
        n221 = call "NCS_Stop.vi"("error in (no error)"=w737, "dosingunit"=3, "device handle in"=w738) -> ("error out"=w735:errorcluster, "device handle out"=w736:u32)
      }
    }
    n222 = case shown="True" "Calibrate 2" {
      tunnel: w201 -> [w719 w724]
      tunnel: w200 -> [w718 w723]
      tunnel: [w719 w722] -> w189
      tunnel: [w718 w721] -> w188
      frame False {
      }
      frame True {
        n223 = call "NCS_Calibrate.vi"("error in (no error)"=w723, "dosingunit"=1, "device handle in"=w724) -> ("error out"=w721:errorcluster, "device handle out"=w722:u32)
      }
    }
    n224 = case shown="True" "Calibrate 3" {
      tunnel: w199 -> [w712 w717]
      tunnel: w198 -> [w711 w716]
      tunnel: [w712 w715] -> w187
      tunnel: [w711 w714] -> w186
      frame False {
      }
      frame True {
        n225 = call "NCS_Calibrate.vi"("error in (no error)"=w716, "dosingunit"=2, "device handle in"=w717) -> ("error out"=w714:errorcluster, "device handle out"=w715:u32)
      }
    }
    n226 = case shown="True" "Calibrate 1" {
      tunnel: w203 -> [w726 w731]
      tunnel: w202 -> [w725 w730]
      tunnel: [w726 w729] -> w191
      tunnel: [w725 w728] -> w190
      frame False {
      }
      frame True {
        n227 = call "NCS_Calibrate.vi"("error in (no error)"=w730, "dosingunit"=0, "device handle in"=w731) -> ("error out"=w728:errorcluster, "device handle out"=w729:u32)
      }
    }
    n228 = case shown="True" "Calibrate 4" {
      tunnel: w197 -> [w705 w710]
      tunnel: w196 -> [w704 w709]
      tunnel: [w705 w708] -> w185
      tunnel: [w704 w707] -> w184
      frame False {
      }
      frame True {
        n229 = call "NCS_Calibrate.vi"("error in (no error)"=w709, "dosingunit"=3, "device handle in"=w710) -> ("error out"=w707:errorcluster, "device handle out"=w708:u32)
      }
    }
    n230 = case shown="True" "Empty 2" {
      tunnel: w189 -> [w685 w689]
      tunnel: w188 -> [w684 w687]
      tunnel: [w685 w688] -> w174
      tunnel: [w684 w686] -> w175
      frame False {
      }
      frame True {
        w691 = 1
        n231 = call "NCS_GetFlowRateMax.vi"("error in (no error)"=w687, "dosingunit"=w691, "device handle in"=w689) -> ("error out"=w692:errorcluster, "flow rate max"=w690:dbl, "device handle out"=w693:u32)
        n232 = call "NCS_EmptySyrige.vi"("error in (no error)"=w692, "flowrate"=w690, "dosingunit"=w691, "device handle in"=w693) -> ("error out"=w686:errorcluster, "device handle out"=w688:u32)
      }
    }
    n233 = case shown="True" "Empty 1" {
      tunnel: w191 -> [w695 w703]
      tunnel: w190 -> [w694 w700]
      tunnel: [w695 w701] -> w172
      tunnel: [w694 w698] -> w173
      frame False {
      }
      frame True {
        w697 = 0
        n234 = call "NCS_GetFlowRateMax.vi"("error in (no error)"=w700, "dosingunit"=w697, "device handle in"=w703) -> ("error out"=w699:errorcluster, "flow rate max"=w696:dbl, "device handle out"=w702:u32)
        n235 = call "NCS_EmptySyrige.vi"("error in (no error)"=w699, "flowrate"=w696, "dosingunit"=w697, "device handle in"=w702) -> ("error out"=w698:errorcluster, "device handle out"=w701:u32)
      }
    }
    n236 = case shown="True" "Empty 3" {
      tunnel: w187 -> [w675 w676]
      tunnel: w186 -> [w674 w677]
      tunnel: [w675 w678] -> w176
      tunnel: [w674 w679] -> w177
      frame False {
      }
      frame True {
        w681 = 2
        n237 = call "NCS_GetFlowRateMax.vi"("error in (no error)"=w677, "dosingunit"=w681, "device handle in"=w676) -> ("error out"=w682:errorcluster, "flow rate max"=w680:dbl, "device handle out"=w683:u32)
        n238 = call "NCS_EmptySyrige.vi"("error in (no error)"=w682, "flowrate"=w680, "dosingunit"=w681, "device handle in"=w683) -> ("error out"=w679:errorcluster, "device handle out"=w678:u32)
      }
    }
    n239 = case shown="True" "Empty 4" {
      tunnel: w185 -> [w665 w666]
      tunnel: w184 -> [w664 w667]
      tunnel: [w665 w669] -> w178
      tunnel: [w664 w668] -> w179
      frame False {
      }
      frame True {
        w671 = 3
        n240 = call "NCS_GetFlowRateMax.vi"("error in (no error)"=w667, "dosingunit"=w671, "device handle in"=w666) -> ("error out"=w672:errorcluster, "flow rate max"=w670:dbl, "device handle out"=w673:u32)
        n241 = call "NCS_EmptySyrige.vi"("error in (no error)"=w672, "flowrate"=w670, "dosingunit"=w671, "device handle in"=w673) -> ("error out"=w668:errorcluster, "device handle out"=w669:u32)
      }
    }
    n242 = Or(x=w114, y="stop") -> (x .or. y?=w130:bool)
    n243 = Or(x=w130, y=w131) -> (x .or. y?=w132:bool)
    n244 = case shown="False" w132 {
      tunnel: [w371 w446] -> w154
      tunnel: [w370 w446] -> w153
      tunnel: [w369 w446] -> w152
      tunnel: [w368 w446] -> w151
      frame False {
        w372 = "?BSI_ReadData"  # ?BSI_ReadData
        n245 = stacked-sequence {
          seq-local: [w373 _ _] -> [_ _ w429]
          tunnel: w372 -> [w373 _ _]
          tunnel: [_ _ w406] -> w371
          tunnel: [_ _ w405] -> w370
          tunnel: [_ _ w404] -> w369
          tunnel: [_ _ w403] -> w368
          frame #0 {
            # "Write Text to Clipboard"
            n246 = String Length(string=w373) -> (length=w382:i32)
            n247 = Increment(x=w382) -> (x+1=w378:i32)
            n248 = dll-call lib="kernel32" fn="GlobalAlloc"("Flags"=i16 0 ("Format"), "Size"=w378) -> (w377:i32)  [unwired: 5 in, 2 out]
            n249 = dll-call lib="kernel32" fn="GlobalLock"("hGlobalMemory"=w377) -> (w380:i32)  [unwired: 4 in, 2 out]
            n250 = dll-call lib="kernel32" fn="lstrcpy"("Flags"=w380, "String"=w373) -> (w379:i32)  [unwired: 5 in, 2 out]
            n251 = stacked-sequence {
              tunnel: w379 -> [_]
              tunnel: w377 -> [w401]
              tunnel: [w400] -> w376
              frame #0 {
                n252 = dll-call lib="kernel32" fn="LocalUnlock"("hGlobalMemory"=w401) -> (w400:i32)  [unwired: 4 in, 2 out]
              }
            }
            "Error Out 2" <- w376
            n253 = case shown="0" w376 {
              selector: w376 -> [_ w397]
              tunnel: w377 -> [w383 _]
              tunnel: [w384 w396] -> w375
              frame 0 {
                n254 = dll-call lib="user32" fn="OpenClipboard"("owner"=i16 0) -> (w385:i32)  [unwired: 4 in, 2 out]
                n255 = case shown="1, Default" w385 {
                  selector: w385 -> [w389 _]
                  tunnel: [w387 w392] -> w384
                  tunnel: w383 -> [_ w391]
                  frame 0 {
                    n256 = Equal To 0?(x=w389) -> (x = 0?=w390:bool)
                    n257 = Bundle(w390, w389, "source"="Error opening clipboard") -> (w387:cluster{bool, i32, "source":string})  [unwired: 1 in]
                  }
                  frame 1, Default {
                    n258 = stacked-sequence {
                      tunnel: [_ _ _ cluster{bool, i32, "source":string} {FALSE, 0, "source"=""} ("Output Element")] -> w392
                      tunnel: w391 -> [_ w393 _ _]
                      frame #0 {
                        n259 = dll-call lib="user32" fn="EmptyClipboard"() -> ()  [unwired: 4 in, 2 out]
                      }
                      frame #1 {
                        n260 = dll-call lib="user32" fn="SetClipboardData"("Format"=1, "Data"=w393) -> ()  [unwired: 6 in, 2 out]
                      }
                      frame #2 {
                        n261 = dll-call lib="user32" fn="CloseClipboard"() -> ()  [unwired: 4 in, 2 out]
                      }
                      frame #3 {
                      }
                    }
                  }
                }
              }
              frame 1, Default {
                n262 = Not Equal To 0?(x=w397) -> (x != 0?=w398:bool)
                n263 = Bundle(w398, w397, "source"="Error copying text to clipboard") -> (w396:cluster{bool, i32, "source":string})  [unwired: 1 in]
              }
            }
            "Write error out 2" <- w375
            n264 = local write "Read Flow Status"("Running" ("Status")) -> ()
          }
          frame #1 {
            # "Wait 500 milliseconds"
            n265 = Wait (ms)(milliseconds to wait=u32 500) -> ()  [unwired: 1 out]
          }
          frame #2 {
            # "Read Text From Clipboard"
            n266 = dll-call lib="user32" fn="OpenClipboard"("owner"=i16 0) -> (w431:i32)  [unwired: 4 in, 2 out]
            n267 = case shown="1, Default" w431 {
              selector: w431 -> [w437 _]
              tunnel: ["" w442] -> w421
              tunnel: [w435 cluster{bool, i32, "source":string} {FALSE, 0, "source"=""} ("Output Element")] -> w430
              frame 0 {
                n268 = Equal To 0?(x=w437) -> (x = 0?=w438:bool)
                n269 = Bundle(w438, w437, "source"="No text in clipboard available!") -> (w435:cluster{bool, i32, "source":string})  [unwired: 1 in]
              }
              frame 1, Default {
                n270 = dll-call lib="user32" fn="GetClipboardData"("uFormat"=1 ("hGlobalMemory")) -> (w443:i32)  [unwired: 4 in, 2 out]
                n271 = dll-call lib="kernel32" fn="GlobalLock"("hGlobalMemory"=w443) -> (w442:string, "hGlobalMemory"=w440:i32)  [unwired: 3 in, 2 out]
                n272 = stacked-sequence {
                  tunnel: w440 -> [w445 _]
                  frame #0 {
                    n273 = dll-call lib="kernel32" fn="LocalUnlock"("hGlobalMemory"=w445) -> ()  [unwired: 5 in, 2 out]
                  }
                  frame #1 {
                    n274 = dll-call lib="user32" fn="CloseClipboard"() -> ()  [unwired: 4 in, 2 out]
                  }
                }
              }
            }
            "Text Read From Clipboard 2" <- w421
            "Read error out 2" <- w430
            n275 = Search/Split String(string=w421, search string/char (-)=" ") -> (substring before match=→"First waste string":string, match + rest of string=w423:string)  [unwired: 1 in, 1 out]
            "Rest of string 1" <- w423
            n276 = Search/Split String(string=w423, search string/char (-)=",") -> (substring before match=w418:string, match + rest of string=w419:string)  [unwired: 1 in, 1 out]
            "First Number" <- w418
            "Rest of string 2" <- w419
            n277 = Search/Split String(string=w419, search string/char (-)="n") -> (substring before match=w416:string, match + rest of string=w409:string)  [unwired: 1 in, 1 out]
            "Second Number 2" <- w416
            "Rest of string 3" <- w409
            n278 = Search/Split String(string=w409, search string/char (-)="i") -> (substring before match=w407:string, match + rest of string=w412:string)  [unwired: 1 in, 1 out]
            "Third Number 3" <- w407
            "Rest of string 4" <- w412
            n279 = Equal?(x=w429, y=w421) -> (x = y?=w428:bool)
            n280 = Search/Split String(string=w412, search string/char (-)="l") -> (substring before match=w410:string, match + rest of string=→"Rest of string 5":string)  [unwired: 1 in, 1 out]
            "Fourth Number 3" <- w410
            n281 = case shown="True" w428 {
              tunnel: ["Response OK" "Failed: No Response from Lab Interface"] -> w427
              frame False {
              }
              frame True {
              }
            }
            "Read Flow Status" <- w427
            n282 = Scan From String(input string=w418) -> (output 1=w406:dbl)  [unwired: 4 in, 3 out]
            "Gas Flow 1 NmL/min" <- w406
            n283 = Scan From String(input string=w416, initial scan location=1) -> (output 1=w405:dbl)  [unwired: 3 in, 3 out]
            "Gas Flow 2 NmL/min" <- w405
            n284 = Scan From String(input string=w407, initial scan location=2) -> (output 1=w404:dbl)  [unwired: 3 in, 3 out]
            "Gas Flow 3 NmL/min" <- w404
            n285 = Scan From String(input string=w410, initial scan location=3) -> (output 1=w403:dbl)  [unwired: 3 in, 3 out]
            "Gas Flow 4 NmL/min" <- w403
            n286 = Merge Signals(w406, w405, w404, w403) -> (→"Gas Flow rate":dynamicdata)
          }
        }
      }
      frame True {
        w446 = 0
      }
    }
    n287 = Merge Signals(w140, w271, w139, w270, w138, w269, w137, w268, w162, w161, w160, w159, w154, w153, w152, w151, w141, w129) -> (w272:dynamicdata)
    n288 = call "Write To Measurement File"("Signals"=w272) -> ()  [unwired: 16 in, 3 out]
    n289 = case shown="True" w130 {
      frame False {
      }
      frame True {
        w309 = "?BSI_SetFlowSetPoints 0,0,0,0,*,*,*,*,*,*,*,*,*,*,*,*,*,*,*,*,*,*,*,*,*,*,*,*,*,*"  # ?BSI_SetFlowSetPoints 0,0,0,0,*,*,*,*,*,*,*,*,*,*,*,*,*,*,*,*,*,*,*,*,*,*,*,*,*,*
        n290 = stacked-sequence {
          seq-local: [w310 _ _] -> [_ _ w343]
          tunnel: w309 -> [w310 _ _]
          frame #0 {
            # "Write Text to Clipboard"
            n291 = String Length(string=w310) -> (length=w319:i32)
            n292 = Increment(x=w319) -> (x+1=w315:i32)
            n293 = dll-call lib="kernel32" fn="GlobalAlloc"("Flags"=i16 0 ("Format"), "Size"=w315) -> (w314:i32)  [unwired: 5 in, 2 out]
            n294 = dll-call lib="kernel32" fn="GlobalLock"("hGlobalMemory"=w314) -> (w317:i32)  [unwired: 4 in, 2 out]
            n295 = dll-call lib="kernel32" fn="lstrcpy"("Flags"=w317, "String"=w310) -> (w316:i32)  [unwired: 5 in, 2 out]
            n296 = stacked-sequence {
              tunnel: w316 -> [_]
              tunnel: w314 -> [w338]
              tunnel: [w337] -> w313
              frame #0 {
                n297 = dll-call lib="kernel32" fn="LocalUnlock"("hGlobalMemory"=w338) -> (w337:i32)  [unwired: 4 in, 2 out]
              }
            }
            "Error Out 5" <- w313
            n298 = case shown="0" w313 {
              selector: w313 -> [_ w334]
              tunnel: w314 -> [w320 _]
              tunnel: [w321 w333] -> w312
              frame 0 {
                n299 = dll-call lib="user32" fn="OpenClipboard"("owner"=i16 0) -> (w322:i32)  [unwired: 4 in, 2 out]
                n300 = case shown="1, Default" w322 {
                  selector: w322 -> [w326 _]
                  tunnel: [w324 w329] -> w321
                  tunnel: w320 -> [_ w328]
                  tunnel: w320 -> [_ _]
                  frame 0 {
                    n301 = Equal To 0?(x=w326) -> (x = 0?=w327:bool)
                    n302 = Bundle(w327, w326, "source"="Error opening clipboard") -> (w324:cluster{bool, i32, "source":string})  [unwired: 1 in]
                  }
                  frame 1, Default {
                    n303 = stacked-sequence {
                      tunnel: [_ _ _ cluster{bool, i32, "source":string} {FALSE, 0, "source"=""} ("Output Element")] -> w329
                      tunnel: w328 -> [_ w330 _ _]
                      frame #0 {
                        n304 = dll-call lib="user32" fn="EmptyClipboard"() -> ()  [unwired: 4 in, 2 out]
                      }
                      frame #1 {
                        n305 = dll-call lib="user32" fn="SetClipboardData"("Format"=1, "Data"=w330) -> ()  [unwired: 6 in, 2 out]
                      }
                      frame #2 {
                        n306 = dll-call lib="user32" fn="CloseClipboard"() -> ()  [unwired: 4 in, 2 out]
                      }
                      frame #3 {
                      }
                    }
                  }
                }
              }
              frame 1, Default {
                n307 = Not Equal To 0?(x=w334) -> (x != 0?=w335:bool)
                n308 = Bundle(w335, w334, "source"="Error copying text to clipboard") -> (w333:cluster{bool, i32, "source":string})  [unwired: 1 in]
              }
            }
            "Write error out 5" <- w312
            n309 = local write "Write Set Point Status 2"("Running" ("Status")) -> ()
          }
          frame #1 {
            # "Wait 500 milliseconds"
            n310 = Wait (ms)(milliseconds to wait=u32 500) -> ()  [unwired: 1 out]
          }
          frame #2 {
            # "Read Text From Clipboard"
            n311 = dll-call lib="user32" fn="OpenClipboard"("owner"=i16 0) -> (w345:i32)  [unwired: 4 in, 2 out]
            n312 = case shown="1, Default" w345 {
              selector: w345 -> [w351 _]
              tunnel: ["" w356] -> w340
              tunnel: [w349 cluster{bool, i32, "source":string} {FALSE, 0, "source"=""} ("Output Element")] -> w344
              frame 0 {
                n313 = Equal To 0?(x=w351) -> (x = 0?=w352:bool)
                n314 = Bundle(w352, w351, "source"="No text in clipboard available!") -> (w349:cluster{bool, i32, "source":string})  [unwired: 1 in]
              }
              frame 1, Default {
                n315 = dll-call lib="user32" fn="GetClipboardData"("uFormat"=1 ("hGlobalMemory")) -> (w357:i32)  [unwired: 4 in, 2 out]
                n316 = dll-call lib="kernel32" fn="GlobalLock"("hGlobalMemory"=w357) -> (w356:string, "hGlobalMemory"=w354:i32)  [unwired: 3 in, 2 out]
                n317 = stacked-sequence {
                  tunnel: w354 -> [w359 _]
                  frame #0 {
                    n318 = dll-call lib="kernel32" fn="LocalUnlock"("hGlobalMemory"=w359) -> ()  [unwired: 5 in, 2 out]
                  }
                  frame #1 {
                    n319 = dll-call lib="user32" fn="CloseClipboard"() -> ()  [unwired: 4 in, 2 out]
                  }
                }
              }
            }
            "Text Read From Clipboard 5" <- w340
            "Read error out 5" <- w344
            n320 = Equal?(x=w343, y=w340) -> (x = y?=w342:bool)
            n321 = case shown="True" w342 {
              tunnel: ["Response OK" "Failed: No Response from Lab Interface"] -> w341
              frame False {
              }
              frame True {
              }
            }
            "Write Set Point Status 2" <- w341
          }
        }
      }
    }
    n322 = case shown="True" "Refill 2" {
      tunnel: w174 -> [w645 w649]
      tunnel: w175 -> [w644 w647]
      tunnel: [w645 w648] -> w170
      tunnel: [w644 w646] -> w165
      frame False {
      }
      frame True {
        w651 = 1
        n323 = call "NCS_GetFlowRateMax.vi"("error in (no error)"=w647, "dosingunit"=w651, "device handle in"=w649) -> ("error out"=w652:errorcluster, "flow rate max"=w650:dbl, "device handle out"=w653:u32)
        n324 = call "NCS_RefillSyrige.vi"("error in (no error)"=w652, "flowrate"=w650, "dosingunit"=w651, "device handle in"=w653) -> ("error out"=w646:errorcluster, "device handle out"=w648:u32)
      }
    }
    n325 = case shown="True" "Refill 1" {
      tunnel: w172 -> [w655 w663]
      tunnel: w173 -> [w654 w660]
      tunnel: [w655 w661] -> w171
      tunnel: [w654 w658] -> w166
      frame False {
      }
      frame True {
        w657 = 0
        n326 = call "NCS_GetFlowRateMax.vi"("error in (no error)"=w660, "dosingunit"=w657, "device handle in"=w663) -> ("error out"=w659:errorcluster, "flow rate max"=w656:dbl, "device handle out"=w662:u32)
        n327 = call "NCS_RefillSyrige.vi"("error in (no error)"=w659, "flowrate"=w656, "dosingunit"=w657, "device handle in"=w662) -> ("error out"=w658:errorcluster, "device handle out"=w661:u32)
      }
    }
    n328 = case shown="True" "Refill 3" {
      tunnel: w176 -> [w635 w636]
      tunnel: w177 -> [w634 w637]
      tunnel: [w635 w638] -> w169
      tunnel: [w634 w639] -> w164
      frame False {
      }
      frame True {
        w641 = 2
        n329 = call "NCS_GetFlowRateMax.vi"("error in (no error)"=w637, "dosingunit"=w641, "device handle in"=w636) -> ("error out"=w642:errorcluster, "flow rate max"=w640:dbl, "device handle out"=w643:u32)
        n330 = call "NCS_RefillSyrige.vi"("error in (no error)"=w642, "flowrate"=w640, "dosingunit"=w641, "device handle in"=w643) -> ("error out"=w639:errorcluster, "device handle out"=w638:u32)
      }
    }
    n331 = case shown="True" "Refill 4" {
      tunnel: w178 -> [w625 w626]
      tunnel: w179 -> [w624 w627]
      tunnel: [w625 w629] -> w168
      tunnel: [w624 w628] -> w163
      frame False {
      }
      frame True {
        w631 = 3
        n332 = call "NCS_GetFlowRateMax.vi"("error in (no error)"=w627, "dosingunit"=w631, "device handle in"=w626) -> ("error out"=w632:errorcluster, "flow rate max"=w630:dbl, "device handle out"=w633:u32)
        n333 = call "NCS_RefillSyrige.vi"("error in (no error)"=w632, "flowrate"=w630, "dosingunit"=w631, "device handle in"=w633) -> ("error out"=w628:errorcluster, "device handle out"=w629:u32)
      }
    }
    n334 = Build Array(w171, w170, w169, w168) -> (w167:u32[])
    n335 = Build Array(w166, w165, w164, w163) -> (w210:errorcluster[])
    "Safety Shut Down Pressure (barg)" <- w133
    "Safety Shut Down Temp (oC)" <- w128
  }
  n336 = call <vilib>:"DAQmx Stop Task.vi"("task/channels in"=w51, "error in"=w50) -> ("task out"=w49:refnum<k21>, "error out"=w48:errorcluster)  [unwired: 12 in]
  n337 = call "CN7500_Write Set Point Value.vi"("Target Set Point Value"=25, "error in (no error)"=w4, "Controller Number"=w1, "VISA In"=w6) -> ("error out"=w3:errorcluster, "VISA Out"=w5:refnum<visa-resource-name>)  [unwired: 6 in]
  n338 = call <vilib>:"DAQmx Clear Task.vi"("task in"=w49, "error in"=w48) -> ()  [unwired: 13 in, 1 out]
  n339 = call "CN7500_Close.vi"("error in (no error)"=w3, "VISA resource name"=w5) -> ()  [unwired: 9 in, 1 out]
  n340 = Index Array(array=w17, index=0) -> (element=w16:u32)
  n341 = Index Array(array=w15, index=0) -> (element=w14:errorcluster)
  n342 = call "NCS_CloseDevice.vi"("error in (no error)"=w14, "device handle"=w16) -> ()  [unwired: 1 out]
